vi "UHR-Fleezers Control (host) - Lorentz v2.vi"() -> ()   [LabVIEW 2014]
uses:
  <vilib>/rvi/interface/nirviMethod/nirviMethod.xnode
  <vilib>/rvi/interface/nirviCloseFPGA/nirviCloseFPGA.xnode
  <vilib>/express/express analysis/Spectral/XNode/ExpressSpectralMeasurementsBlockNode.xnode
  <vilib>/rvi/interface/nirviReadWriteControl/nirviReadWriteControl.xnode
  <vilib>/Analysis/NI_AALBase.lvlib
  <vilib>/express/express analysis/Spectral/Block/exnSpectralBlock spectral measurements PSD poly.vi
  <vilib>/rvi/interface/nirviOpenFPGA/nirviOpenFPGA.xnode
  <vilib>/Platform/TimedLoop/XDataNode/XDataNode.xnode
  <vilib>/Platform/TimedLoop/XDataNode/nitl_modes.ctl
  <vilib>/Platform/TimedLoop/XDataNode/XDNodeRunTimeDep.lvlib
  <vilib>/Platform/TimedLoop/XDataNode/wakeup.ctl
  <vilib>/Platform/TimedLoop/XDataNode/timing_clust.ctl
  <vilib>/Utility/miscctls.llb/LVPoint32TypeDef.ctl
  <vilib>/userdefined/High Color/nirio_resource_hc.ctl
  openfpgaref.8.6.ctl
  <vilib>/Utility/miscctls.llb/LVMinMaxIncTypeDef.ctl
  <vilib>/Instr/_visa.llb/VISA Configure Serial Port (Instr).vi
  <vilib>/Analysis/baseanly.llb/Mean (DBL).vi
  Duncan Nall/Fluorescence simulation/Global for fluorescence simulation mean (30 samples), (power series).vi
  <vilib>/vision/Avi.llb/IMAQ AVI2 Refnum.ctl
  <vilib>/gmath/NI_Gmath.lvlib
  <vilib>/addons/database/NI_Database_API.lvlib
  uFLUX control_v2/uFLUX control_v2/Pressure Control/Pressure Control.lvclass
  uFLUX control_v2/uFLUX control_v2/TTL/TTL.lvclass
  uFLUX control_v2/uFLUX control_v2/Pressure Control/Pressure Control Config.ctl
  <vilib>/rvi/errors/niLvFpgaMergeErrorWithErrorCode.vi
  UHR-Fleezers Control (fpga) - Lorentz 1.vi
  <vilib>/addons/database/Connection.llb/DB Tools Open Connec (Path).vi
  <vilib>/Waveform/WDTOps.llb/WDT Index Channel DBL.vi
  <vilib>/Waveform/WDTOps.llb/WDT Append Waveforms DBL.vi
  <vilib>/sound2/lvsound2.llb/Sound Output Write (DBL Single).vi
  <vilib>/express/express analysis/Spectral/Block/exnSpectralBlock spectral measurements PSD WFM.vi
  FPGA Bitfiles/UHR-FleezersInst_FPGATarget_UHR-FleezersCont_eGrpOyvbXfI.lvbitx
  <vilib>/addons/database/Connection.llb/Conn ObjectReference.ctl
  <vilib>/sound2/lvsound2.llb/Sampling Mode.ctl
  <vilib>/sound2/lvsound2.llb/Sound Data Format.ctl
panel:
  in  "Save Event Log?":bool=TRUE
  in  "Stop saving data + video":bool
  in  "Start saving data + video":bool
  in  "Bead diameter":dbl=800.0
  in  "Channel 1 Buffer":string
  in  "DNA Construct":string="oligo binding"
  in  "Title":string="testing database"
  in  "Name":string="test name"
  out "Total Time (s) 2":dbl=60.0
  in  "Start Saving":bool
  in  "Comment (data description)":string="testing confocal setup"
  out "Calibrating Trap...":bool
  in  "N sets to save":u32=200 caption="N Sets"
  in  "Save N Sets":bool
  out "Save file name":path=path "P:/Data/160111/160111_031.dat"
  in  "Save ave N":dbl=100.0 caption="Averaging Factor"
  out "Saving...":bool
  in  "Stop Saving":bool
  out "Progress":u16(slide) scale=0.0..100.0
  out "Save Data Rate (Hz)":dbl=666.6666666666667 caption="Rate (Hz)" format="%#_6p"
  out "Save Data Period (s)":dbl=0.0014999999999999998 caption="Period (s)" format="%#_6p"
  in  "Channel 2 Buffer":string="NA"
  in  "Channel 3 Buffer":string="NA"
  out "Read offset current":string(combo)
  out "PSD Y Sum":dbl[](array[numeric])
  out "log file ref":refnum<file>
  out "AL Running":bool
  in  "AL Delay (s)":u32
  in  "Stop assembly line":bool
  in  "Cy5 Fl.  Thresh. (kHz)":dbl=24.5
  in  "Cy3 Fl.  Thresh. (kHz)":dbl=19.0
  in  "Get Fluorophore":bool
  in  "X or Y?":bool=TRUE
  out "Red Fluorophore":bool
  out "Green Fluorophore":bool
  in  "Numeric":dbl
  in  "stop":bool
  in  "Start assembly line":bool
  out "Sigma/Mean 3":dbl=nan caption="Sigma/Mean" format="%#_2g"
  out "Rate sigma (Hz) 3":dbl=-0.0 caption="Sigma (Hz)" format="%0.2f"
  out "APD 3 Rate (Hz)":dbl=nan format="%#_3p"
  out "HP3 Flush Time (s)":dbl=90.0
  out "HP1 Flush Time (s)":dbl=60.0
  out "TTrig":cluster{dbl, dbl}(graph)
  in  "Sample Channel\nFlow":bool
  in  "Inject Pump 1":bool
  in  "Inject Pump 3":bool
  in  "Pump 1 contents":string="Bottom: DNA beads" caption="Contents"
  in  "Pump 3 contents":string="Top: ADig beads" caption="Contents"
  out "Time (s)":dbl=5.700284999999999
  in  "Index":dbl=1.0 caption="Save File Index" min=1.0 step=1.0
  in  "Scripts":T1(tab)
  in  "Calibrate after bead 2?":bool
  in  "Number of Pulses for bead 2":i32
  in  "Number of pulses for Bead 1":i32
  in  "Get New Beads":bool
  in  "Fixed Traps Data\nScript":bool
  in  "Dump spot flow on?":bool=TRUE caption="Flow ON?"
  in  "Daq spot flow on":bool=TRUE caption="Flow ON?"
  in  "Cap 1 Samp Flow ON":bool=TRUE
  in  "Cap 2 Samp Flow ON":bool=TRUE
  in  "Got Bead 2":bool
  in  "Got Bead 1":bool
  in  "Cap 2 Flow ON":bool=TRUE
  in  "Cap 1 Flow ON":bool=TRUE
  in  "Cap 2 T ON":bool=TRUE
  in  "Move Cap. 2 (ADig Top)":bool
  in  "Move Cap. 1 (DNA Bottom)":bool
  in  "Cal/Data Acq. Spot":bool
  in  "Dump Beads":bool
  in  "Cap 1 T ON":bool=TRUE
  in  "Force FB Data\nScript":bool
  in  "Cap. 2 BD T1?\n(ADig T1, DNA T2)":bool
  in  "Flow Cal":bool
  in  "Pulse Duration (0-100 ms)":dbl=10.0
  in  "Number of pulses For laminar flow":i32=1
  in  "Vent pressure":bool=TRUE
  in  "Pressure Up":bool=TRUE
  in  "Pressure Down":bool=TRUE
  in  "Active cal after cal?":bool
  in  "Fish after cal?":bool
  in  "Flow ON during cal?":bool
  in  "Offset 2 Set":dbl=2.0
  in  "Offset 1 Set":dbl
  in  "Cal @ (MHz)":dbl=14.0
  in  "W/ Offset 1":bool=TRUE
  in  "Offset 1 Start (MHz)":dbl=10.0
  in  "W/ Offset 2":bool
  in  "Offset 2 Start (MHz)":dbl=16.0
  in  "Cal Stage Position":i32=3
  in  "Flow based calibration?":bool
  in  "Lumicks Flow During Calibration":bool
  in  "Only check fixed trap T2":bool
  in  "Flow ON after\ntether testing?":bool
  in  "Flow ON during \nfishing?":bool
  in  "Fish again after \nraster break?":bool
  in  "Furthest Delta (MHz)":dbl=15.0 step=0.25
  in  "Green ON During Raster":bool
  in  "Move to Delta 2 (MHz)":dbl=12.3
  in  "Attempt Limit":dbl=20.0 caption="Limit"
  out "Attempts":dbl=10.0
  in  "Wait Before Save (s)":u32=1
  in  "Closest Delta (MHz)":dbl=8.0 step=0.25
  in  "Stop F (pN)":dbl=3.0
  in  "Then...":string(combo)="5"
  in  "Move to Delta 1 (MHz)":dbl=10.0
  in  "Tether Alarm?":bool=TRUE
  out "Tether":bool
  in  "TA Cancel Save?":bool
  in  "TA Green Off?":bool
  in  "Raster Set Upon Tether":u32=5
  in  "Save at end (5, 6)":bool
  in  "Stop Fishing When Tether":bool=TRUE
  in  "Delay before dipping (s)":dbl=5.0
  in  "Start dipping after?":bool
  in  "Green ON after FB ON?":bool
  in  "Remove Action Offset":bool
  in  "Stage Position To Establish FB":i32=3
  in  "Trap Trig Fl.":bool
  in  "Starting \nTrap Delta (MHz)":dbl=15.25
  in  "Trap Delta Before Moving":dbl=13.0
  in  "Wait (s)":u32=1
  in  "Green ON":bool
  in  "Start dipping after?":bool=TRUE
  in  "Fixed Traps Trap Delta (MHz)":dbl=15.25 caption="Trap Delta (MHz)"
  out "TTrig Fin Thresh (nm)":dbl
  out "TTrig Sig (nm)":dbl
  out "Threshold stored (nm)":dbl
  in  "Neg. TTrig FPGA":bool=TRUE
  in  "Test ttrig":bool
  in  "Trap Trig. (FPGA)":bool=TRUE
  out "Initializing":bool
  in  "Reinitialize":bool
  out "Triggered":bool
  out "Waiting":bool
  in  "Trap Trig. Fl.":bool
  in  "Wait to get offset (n)":u32=10
  in  "Threshold (nm)":dbl=15.0
  in  "Fl. ON time (n)":i32=90
  out "T1 x pos data":dbl[](array[numeric])
  out "max value":dbl=-0.9003514563721442
  out "min value":dbl=-1.184251119672945
  in  "Mean T1 Position\nto compare (nm)":dbl caption="Mean T1 for Comparison (nm)" format="%0.2f"
  out "mean":dbl=-1.0423012880225446 format="%0.2f"
  out "standard\ndeviation":dbl=0.2007473770965739 format="%0.2f"
  out "TTrig Sig (Int)":i64
  out "TTrig Fin Thresh (Int)":i64
  in  "FB Trig Integrate":u32=1
  in  "Green ON\nafter start\nreturn?":bool
  in  "Green delay after \nstart return (s)":dbl
  out "Dwell Time (s)":dbl
  in  "FB OFF when \nflow ON":bool
  in  "Flow ON \nduring return\nfrom dip?":bool=TRUE
  in  "Flow ON\nduring daq?":bool=TRUE
  in  "Flow ON\nduring dip?":bool=TRUE
  in  "Cancel dwell":bool
  in  "Pause dwell":bool
  in  "Dwell Duration (s)":i32=45
  in  "Green ON\nbefore dip?":bool
  in  "Cont. Repeat Dipping?":bool=TRUE
  in  "Dipping Delta (MHz)":dbl=15.0
  in  "Move trap \nbefore dip move?":bool
  in  "Save data after return?":bool
  in  "Green ON \nafter return?":bool=TRUE
  in  "Dip Trap Delta 2 (MHz)":dbl=15.0
  in  "Move trap after return?":bool
  in  "Dip Duration (s)":i32=15
  in  "Dip for Protein":bool
  in  "Dip Stage \nPosition":i32=5
  in  "Return Stage \nPosition":i32=3
  out "Dip Time (s)":i32=16
  out "Dip #":i32=5
  in  "Y change (mm)":dbl=-3.0
  in  "Profile":bool
  out "Current Position":cluster{dbl, dbl, dbl}={1.6, 0.50781, -0.0311}
  in  "Shift confocal":bool
  in  "Auto F Reset":bool
  in  "Yank when?":bool
  in  "Yank to which?":bool
  in  "Yank to SP":dbl[](array[numeric])=[-0.128, -0.158, -0.183, -0.21, -0.01, -0.0319, -0.094, -0.143]
  in  "APD to Watch":bool
  out "Duration (s)":dbl=8.399999999999977
  in  "Action":string(combo)="Yank"
  in  "Fl. Triggered...":bool
  in  "Fl. Delta Thresh. (kHz)":dbl=0.14
  out "Waiting":bool
  out "Fl. High":bool
  in  "N pts to average":u16=6
  in  "Yank Delay (s)":dbl=3.0
  in  "Yank to Trap Delta (MHz)":dbl[](array[numeric])=[16.3, 15.85, 14.85]
  in  "N Array El":u8=4 min=1 step=1
  in  "Random Choice":bool=TRUE
  in  "Force Yank":bool
  in  "Reset Force":bool
  in  "N Steps":dbl=20.0
  in  "Step Size (nm)":dbl=0.34
  in  "Save ave factor":dbl=1.0
  in  "Take Stepping Data":bool
  out "Sigma/Mean 2":dbl=nan caption="Sigma/Mean" format="%#_2g"
  out "Rate sigma (Hz) 2":dbl=-0.0 caption="Sigma (Hz)" format="%0.2f"
  out "APD 2 Rate (Hz)":dbl=nan format="%#_3p"
  out "Primary Video Display":T2(plugin-control)
  out "Waveform Graph":dbl[](graph)=[25.0, 1151.0, 841.0, 408.0, 301.0, 290.0, 352.0, 294.0, 340.0, 282.0, 211.0, 161.0, 111.0, 35.0, 21.0, 13.0, 7.0, 8.0, 6.0, 2.0, 6.0, 11.0, 2.0, 3.0, 7.0, 8.0, 12.0, 13.0, 20.0, 53.0, 62.0, 57.0, 60.0, 49.0, 37.0, 25.0, 16.0, 5.0, 4.0, 4.0, 1.0, 1.0, 1.0, 4.0, 7.0, 9.0, 12.0, 16.0, 28.0, 31.0, 50.0, 54.0, 55.0, 47.0, 50.0, 30.0, 9.0, 10.0, 4.0, 3.0, 3.0, 0.0, 1.0, 2.0, 1.0, 3.0, 9.0, 10.0, 32.0, 32.0, 86.0, 115.0, 183.0, 243.0, 350.0, 369.0, 337.0, 307.0, 224.0, 155.0] caption="APD Line Scan"
  out "Messages":string="14:51\tUHR-Fleezers ready.\r"
  in  "APD Ave N":dbl=20.0
  out "Int. Time (s)":dbl
  in  "Stop All":bool=TRUE
  out "Sigma/Mean":dbl=nan format="%#_2g"
  out "Rate sigma (Hz)":dbl=-0.0 caption="Sigma (Hz)" format="%0.2f"
  in  "Tab Control 6":T3(tab)
  in  "APD 3 Offset":dbl
  in  "APD 2 Offset":dbl
  in  "APD 1 Offset":dbl
  out "RMS (Ang)":dbl=nan format="%_2g"
  in  "Bead Sep. Int. Time (s)":dbl=3.0 caption="Int. Time (s)"
  in  "Below (kHz)":dbl=1.0
  in  "Above (kHz)":dbl=2.0
  in  "Adjust Scale\nto Mean":bool
  in  "Remove Offset":bool
  in  "Offset (nm)":dbl format="%#_3g"
  out "Mean":dbl=nan caption="Mean (pN)" format="%#_3g"
  out "Force":waveform(dbl)[](graph)=[{"t0"=timestamp(0 s since 1904-01-01), "dt"=0.15, "Y"=[], "attributes"=variant("NI_ChannelName"=variant(string "T1 X"))}, {"t0"=timestamp(0 s since 1904-01-01), "dt"=0.15, "Y"=[], "attributes"=variant("NI_ChannelName"=variant(string "T2 X"))}, {"t0"=timestamp(0 s since 1904-01-01), "dt"=0.15, "Y"=[], "attributes"=variant("NI_ChannelName"=variant(string "T1 X"))}]
  out "APD Chart":waveform(dbl)[](graph)=[{"t0"=timestamp(0 s since 1904-01-01), "dt"=0.15, "Y"=[], "attributes"=variant("NI_ChannelName"=variant(string "APD 1"))}, {"t0"=timestamp(0 s since 1904-01-01), "dt"=0.15, "Y"=[], "attributes"=variant("NI_ChannelName"=variant(string "APD 2"))}, {"t0"=timestamp(0 s since 1904-01-01), "dt"=0.15, "Y"=[], "attributes"=variant("NI_ChannelName"=variant(string "APD 3"))}]
  in  "Calibration":u16(ring)=2 items=["None", "Position", "Force"]
  out "T1 X":dbl=nan caption="T1 X (pN)" format="%0.2f"
  out "T2 X":dbl=nan caption="T2 X (pN)" format="%0.2f"
  out "Bead Separation":waveform(dbl)(graph)={"t0"=timestamp(0 s since 1904-01-01), "dt"=0.15, "Y"=[], "attributes"=variant("NI_ChannelName"=variant(string "T1 X"))}
  out "Bead Mean (nm)":dbl=nan caption="Mean (nm)" format="%0.2f"
  out "Difference":dbl=nan caption="Difference (pN)" format="%.2g"
  out "Confocal Y 2 (V)":dbl=6.809280068361465
  out "Confocal X 2 (V)":dbl=0.7223435163426621
  out "Confocal Y 1 (V)":dbl=5.709081392864773
  out "Confocal X 1 (V)":dbl=4.827825251014741
  in  "Set High F Confocal Spot (X-Y)":bool
  in  "Take Detection Laser\nImage":bool
  out "APD 2":T2(plugin-control) caption="APD 2 (Cy5)"
  in  "Flip Green Filter":bool
  in  "Set X Only":bool
  in  "Set Y Only":bool
  out "APD 1":T2(plugin-control) caption="APD 1 (Cy3)"
  out "Detection Laser Y":T2(plugin-control)
  out "Pointer Y (V)":dbl=4.837472762230294 format="%_3g"
  out "Pointer X (V)":dbl=8.31425977355266 format="%_3g"
  in  "Set Confocal Spot (X-Y)":bool
  out "Detection Laser X":T2(plugin-control)
  out "APD 3":T2(plugin-control) caption="APD 3 (Cy2)"
  in  "Display Saved Data":string(combo)
  out "Saved trap pos":dbl[](graph)
  out "Saved APD":dbl[][](graph)=[[126.66666666666667, 113.33333333333334, 126.66666666666667, 113.33333333333334, 80.0, 133.33333333333334, 53.333333333333336, 106.66666666666667, 86.66666666666667, 53.333333333333336, 80.0, 160.0, 113.33333333333334, 100.0, 120.0, 153.33333333333334, 140.0, 93.33333333333334, 106.66666666666667, 133.33333333333334, 113.33333333333334, 100.0, 126.66666666666667, 140.0, 153.33333333333334, 100.0, 60.0, 120.0, 86.66666666666667, 80.0, 100.0, 73.33333333333334, 86.66666666666667, 113.33333333333334, 60.0, 126.66666666666667, 113.33333333333334, 100.0, 113.33333333333334, 113.33333333333334, 93.33333333333334, 86.66666666666667, 146.66666666666669, 86.66666666666667, 126.66666666666667, 80.0, 113.33333333333334, 153.33333333333334, 86.66666666666667, 60.0, 86.66666666666667, 106.66666666666667, 113.33333333333334, 106.66666666666667, 133.33333333333334, 133.33333333333334, 53.333333333333336, 146.66666666666669, 153.33333333333334, 80.0, 73.33333333333334, 113.33333333333334, 100.0, 113.33333333333334, 120.0, 86.66666666666667, 86.66666666666667, 93.33333333333334, 60.0, 80.0, 120.0, 126.66666666666667, 46.66666666666667, 173.33333333333334, 113.33333333333334, 66.66666666666667, 140.0, 113.33333333333334, 53.333333333333336, 86.66666666666667, 46.66666666666667, 80.0, 113.33333333333334, 126.66666666666667, 100.0, 60.0, 93.33333333333334, 80.0, 106.66666666666667, 140.0, 113.33333333333334, 140.0, 93.33333333333334, 106.66666666666667, 93.33333333333334, 86.66666666666667, 140.0, 133.33333333333334, 1760.0, 3533.3333333333335, 380.0, 4466.666666666667, 5073.333333333334, 826.6666666666667, 6466.666666666667, 2680.0, 4713.333333333334, 8260.0, 1026.6666666666667, 8900.0, 8820.0, 1940.0, 10873.333333333334, 4460.0, 5406.666666666667, 9986.666666666668, 1446.6666666666667, 9040.0, 6800.0, 1920.0, 7273.333333333334, 3226.666666666667, 3053.3333333333335, 5526.666666666667, 753.3333333333334, 3440.0, 2600.0, 726.6666666666667, 1993.3333333333335, 973.3333333333334, 0.0, 0.0, 6.666666666666667, 20.0, 6.666666666666667, 0.0, 0.0, 13.333333333333334, 0.0, 13.333333333333334, 6.666666666666667, 0.0, 0.0, 6.666666666666667, 6.666666666666667, 6.666666666666667, 6.666666666666667, 20.0, 0.0, 6.666666666666667, 0.0, 6.666666666666667, 6.666666666666667, 0.0, 0.0, 0.0, 0.0, 0.0, 6.666666666666667, 6.666666666666667, 0.0, 6.666666666666667, 58873.333333333336, 88753.33333333334, 58686.66666666667, 82013.33333333334, 73680.0, 86226.66666666667, 161553.33333333334, 90873.33333333334, 99960.0, 160820.0, 143406.6666666667, 123873.33333333334, 111920.0, 138946.6666666667, 203493.33333333334, 115073.33333333334, 113620.0, 165526.6666666667, 162766.6666666667, 108720.0, 105680.0, 128066.66666666667, 161266.6666666667, 91606.66666666667, 81740.0, 105920.0, 114013.33333333334, 57840.0, 56013.333333333336, 49453.333333333336, 55046.66666666667, 24753.333333333336, 37073.333333333336, 59220.0, 40473.333333333336, 53360.0, 48266.66666666667, 57626.66666666667, 113800.0, 64993.333333333336, 76386.66666666667, 121100.0, 109613.33333333334, 93006.66666666667, 87486.66666666667, 109153.33333333334, 161280.0, 91160.0, 90606.66666666667, 134300.0, 129660.0, 88133.33333333334, 85346.66666666667, 100960.0, 129826.66666666667, 74526.66666666667, 63600.0, 86580.0, 90173.33333333334, 43646.66666666667, 42160.0, 37413.333333333336, 39540.0, 16886.666666666668, 83180.0, 145886.6666666667, 135013.33333333334, 143420.0, 131746.6666666667, 171326.6666666667, 260526.6666666667, 152053.33333333334, 159300.0, 237413.33333333334, 234720.0, 179213.33333333334, 168473.33333333334, 213053.33333333334, 275106.6666666667, 166913.33333333334, 163233.33333333334, 234900.0, 240626.6666666667, 161813.33333333334, 156160.0, 194220.0, 241986.6666666667, 141060.0, 130106.66666666667, 178380.0, 181720.0, 101760.0, 97240.0, 91920.0, 106166.66666666667, 53620.0, 49766.66666666667, 69306.66666666667, 76120.0, 85406.66666666667, 80873.33333333334, 111693.33333333334, 191113.33333333334, 113333.33333333334, 122166.66666666667, 187080.0, 194293.33333333334, 142746.6666666667, 138233.33333333334, 178420.0, 243293.33333333334, 143806.6666666667, 139293.33333333334, 202140.0, 213406.6666666667, 138013.33333333334, 136020.0, 165513.33333333334, 212093.33333333334, 120806.66666666667, 109833.33333333334, 149353.33333333334, 148793.33333333334, 77393.33333333334, 77113.33333333334, 69493.33333333334, 77660.0, 33440.0, 50560.0, 68646.66666666667, 74726.66666666667, 84220.0, 78213.33333333334, 109353.33333333334, 188906.6666666667, 110473.33333333334, 123720.0, 187960.0, 194106.6666666667, 144266.6666666667, 138713.33333333334, 174200.0, 242460.0, 143686.6666666667, 141326.6666666667, 201426.6666666667, 211853.33333333334, 138133.33333333334, 136433.33333333334, 162713.33333333334, 215760.0, 122100.0, 109560.0, 151720.0, 151620.0, 78946.66666666667, 79433.33333333334, 68566.66666666667, 82966.66666666667, 37260.0, 14106.666666666668, 13780.0, 19180.0, 19686.666666666668, 20360.0, 33320.0, 69573.33333333334, 39166.66666666667, 48846.66666666667, 84226.66666666667, 91106.66666666667, 62666.66666666667, 58206.66666666667, 74120.0, 110460.0, 58186.66666666667, 61666.66666666667, 88013.33333333334, 91280.0, 58646.66666666667, 58420.0, 65173.333333333336, 87826.66666666667, 47933.333333333336, 41393.333333333336, 49720.0, 50586.66666666667, 20986.666666666668, 21160.0, 13453.333333333334, 16726.666666666668, 6206.666666666667, 67173.33333333334, 100193.33333333334, 104320.0, 110186.66666666667, 103286.66666666667, 139606.6666666667, 222940.0, 130420.0, 139753.33333333334, 209046.6666666667, 211860.0, 159173.33333333334, 152006.6666666667, 192673.33333333334, 259866.6666666667, 154100.0, 153553.33333333334, 217093.33333333334, 223493.33333333334, 147993.33333333334, 144046.6666666667, 177720.0, 223973.33333333334, 129053.33333333334, 117240.0, 159020.0, 157046.6666666667, 83680.0, 79880.0, 72200.0, 86860.0, 38986.66666666667, 11033.333333333334, 11433.333333333334, 18180.0, 21460.0, 19020.0, 35926.66666666667, 65173.333333333336, 37820.0, 45606.66666666667, 70533.33333333334, 83633.33333333334, 50833.333333333336, 52286.66666666667, 69380.0, 100033.33333333334, 57246.66666666667, 50233.333333333336, 73880.0, 81306.66666666667, 52020.0, 50640.0, 64780.0, 78986.66666666667, 45466.66666666667, 35400.0, 47693.333333333336, 45946.66666666667, 18393.333333333336, 16966.666666666668, 12926.666666666668, 15080.0, 5193.333333333334, 7446.666666666667, 7086.666666666667, 13886.666666666668, 14406.666666666668, 15820.0, 27906.666666666668, 45180.0, 27386.666666666668, 31680.0, 45973.333333333336, 65326.66666666667, 42586.66666666667, 42646.66666666667, 59326.66666666667, 73720.0, 44526.66666666667, 39353.333333333336, 56040.0, 66106.66666666667, 40246.66666666667, 39933.333333333336, 54113.333333333336, 59526.66666666667, 33786.66666666667, 27826.666666666668, 33466.66666666667, 38540.0, 14500.0, 13646.666666666668, 11393.333333333334, 10433.333333333334, 3666.666666666667, 7286.666666666667, 7800.0, 11813.333333333334, 14140.0, 14900.0, 25013.333333333336, 44160.0, 27293.333333333336, 34553.333333333336, 47473.333333333336, 64253.333333333336, 38960.0, 41173.333333333336, 51546.66666666667, 64260.0, 38813.333333333336, 37706.66666666667, 52513.333333333336, 61353.333333333336, 36746.66666666667, 34513.333333333336, 44786.66666666667, 49726.66666666667, 28846.666666666668, 21580.0, 30246.666666666668, 30433.333333333336, 12300.0, 11606.666666666668, 8053.333333333334, 6646.666666666667, 3166.666666666667, 7313.333333333334, 6826.666666666667, 9246.666666666668, 12060.0, 10813.333333333334, 21320.0, 39206.66666666667, 24040.0, 28600.0, 42253.333333333336, 59766.66666666667, 31160.0, 34020.0, 43793.333333333336, 54166.66666666667, 33813.333333333336, 33253.333333333336, 39600.0, 51773.333333333336, 31746.666666666668, 29406.666666666668, 39226.66666666667, 43393.333333333336, 25960.0, 21453.333333333336, 25940.0, 32280.0, 12853.333333333334, 10880.0, 7473.333333333334, 7173.333333333334, 2920.0, 56953.333333333336, 85960.0, 58406.66666666667, 90333.33333333334, 84813.33333333334, 120433.33333333334, 207333.33333333334, 121233.33333333334, 137100.0, 211380.0, 212946.6666666667, 175960.0, 158733.33333333334, 214973.33333333334, 269733.3333333334, 169720.0, 163193.33333333334, 235040.0, 255906.6666666667, 166186.6666666667, 159446.6666666667, 215633.33333333334, 244666.6666666667, 153406.6666666667, 147000.0, 191020.0, 219800.0, 124920.0, 124533.33333333334, 147293.33333333334, 157046.6666666667, 88060.0, 54086.66666666667, 70540.0, 76433.33333333334, 81826.66666666667, 85986.66666666667, 113520.0, 176380.0, 112013.33333333334, 123620.0, 173073.33333333334, 198520.0, 139326.6666666667, 135673.33333333334, 187406.6666666667, 227553.33333333334, 144433.33333333334, 140100.0, 190633.33333333334, 223760.0, 137513.33333333334, 134286.6666666667, 176153.33333333334, 199046.6666666667, 119846.66666666667, 108193.33333333334, 137506.6666666667, 160513.33333333334, 75686.66666666667, 77973.33333333334, 74446.66666666667, 71320.0, 34140.0, 35486.66666666667, 47333.333333333336, 55853.333333333336, 61040.0, 57560.0, 86853.33333333334, 140953.33333333334, 90080.0, 99880.0, 142580.0, 178360.0, 121720.0, 121386.66666666667, 156453.33333333334, 196960.0, 125066.66666666667, 121120.0, 169926.6666666667, 196686.6666666667, 121786.66666666667, 118093.33333333334, 158286.6666666667, 173840.0, 106106.66666666667, 95486.66666666667, 115780.0, 135840.0, 60906.66666666667, 60800.0, 53900.0, 55026.66666666667, 26106.666666666668, 48733.333333333336, 70033.33333333334, 9786.666666666668, 97153.33333333334, 106946.66666666667, 50066.66666666667, 162993.33333333334, 135240.0, 169180.0, 240760.0, 115480.0, 279280.0, 243513.33333333334, 170540.0, 246993.33333333334, 239593.33333333334, 217593.33333333334, 267820.0, 139560.0, 262060.0, 222146.6666666667, 136953.33333333334, 206126.6666666667, 159126.6666666667, 109660.0, 153573.33333333334, 16346.666666666668, 100873.33333333334, 53153.333333333336, 9793.333333333334, 29960.0, 11113.333333333334, 36153.333333333336, 44553.333333333336, 9400.0, 65753.33333333334, 72673.33333333334, 46580.0, 121946.66666666667, 122980.0, 150580.0, 206953.33333333334, 111460.0, 250006.6666666667, 218440.0, 173186.6666666667, 227593.33333333334, 227180.0, 205006.6666666667, 243653.33333333334, 130620.0, 242040.0, 198446.6666666667, 133746.6666666667, 186313.33333333334, 140640.0, 91306.66666666667, 124153.33333333334, 15173.333333333334, 76546.66666666667, 35246.66666666667, 8000.0, 18240.0, 6306.666666666667, 100.0, 53.333333333333336, 46.66666666666667, 73.33333333333334, 93.33333333333334, 60.0, 40.0, 53.333333333333336, 106.66666666666667, 106.66666666666667, 60.0, 93.33333333333334, 66.66666666666667, 66.66666666666667, 73.33333333333334, 66.66666666666667, 73.33333333333334, 40.0, 53.333333333333336, 93.33333333333334, 46.66666666666667, 33.333333333333336, 66.66666666666667, 80.0, 33.333333333333336, 73.33333333333334, 80.0, 53.333333333333336, 33.333333333333336, 60.0, 73.33333333333334, 66.66666666666667, 73.33333333333334, 60.0, 106.66666666666667, 80.0, 80.0, 46.66666666666667, 66.66666666666667, 126.66666666666667, 46.66666666666667, 26.666666666666668, 46.66666666666667, 33.333333333333336, 66.66666666666667, 93.33333333333334, 73.33333333333334, 66.66666666666667, 73.33333333333334, 60.0, 53.333333333333336, 80.0, 33.333333333333336, 60.0, 100.0, 80.0, 80.0, 73.33333333333334, 73.33333333333334, 126.66666666666667, 46.66666666666667, 106.66666666666667, 106.66666666666667, 120.0, 113.33333333333334, 93.33333333333334, 93.33333333333334, 66.66666666666667, 100.0, 120.0, 53.333333333333336, 113.33333333333334, 133.33333333333334, 140.0, 53.333333333333336, 160.0, 160.0, 106.66666666666667, 113.33333333333334, 66.66666666666667, 106.66666666666667, 106.66666666666667, 100.0, 146.66666666666669, 173.33333333333334, 120.0, 93.33333333333334, 153.33333333333334, 113.33333333333334, 126.66666666666667, 100.0, 133.33333333333334, 146.66666666666669, 180.0, 126.66666666666667, 126.66666666666667, 126.66666666666667, 93.33333333333334, 126.66666666666667, 93.33333333333334, 120.0, 80.0, 93.33333333333334, 100.0, 73.33333333333334, 146.66666666666669, 100.0, 46.66666666666667, 53.333333333333336, 40.0, 73.33333333333334, 60.0, 80.0, 80.0, 66.66666666666667, 60.0, 53.333333333333336, 80.0, 86.66666666666667, 33.333333333333336, 66.66666666666667, 73.33333333333334, 86.66666666666667, 73.33333333333334, 53.333333333333336, 66.66666666666667, 66.66666666666667, 73.33333333333334, 40.0, 100.0, 46.66666666666667, 46.66666666666667, 86.66666666666667, 53.333333333333336, 66.66666666666667, 60.0, 93.33333333333334, 73.33333333333334, 60.0, 86.66666666666667, 53.333333333333336, 53.333333333333336, 86.66666666666667, 53.333333333333336, 66.66666666666667, 66.66666666666667, 66.66666666666667, 60.0, 100.0, 40.0, 60.0, 40.0, 46.66666666666667, 73.33333333333334, 53.333333333333336, 60.0, 86.66666666666667, 86.66666666666667, 60.0, 46.66666666666667, 33.333333333333336, 86.66666666666667, 106.66666666666667, 60.0, 40.0, 86.66666666666667, 66.66666666666667, 53.333333333333336, 46.66666666666667, 86.66666666666667, 13.333333333333334, 53.333333333333336, 73.33333333333334, 46.66666666666667, 53.333333333333336, 80.0, 86.66666666666667, 40.0, 100.0, 86.66666666666667, 80.0, 53.333333333333336, 66.66666666666667, 60.0, 60.0, 113.33333333333334, 60.0, 60.0, 53.333333333333336, 100.0, 80.0, 53.333333333333336, 73.33333333333334, 86.66666666666667, 73.33333333333334, 53.333333333333336, 73.33333333333334, 113.33333333333334, 100.0, 80.0, 66.66666666666667, 66.66666666666667, 53.333333333333336, 60.0, 86.66666666666667, 73.33333333333334, 120.0, 106.66666666666667, 73.33333333333334, 40.0, 120.0, 86.66666666666667, 66.66666666666667, 113.33333333333334, 120.0, 106.66666666666667, 126.66666666666667, 133.33333333333334, 93.33333333333334, 113.33333333333334, 120.0, 86.66666666666667, 100.0, 106.66666666666667, 160.0, 86.66666666666667, 100.0, 93.33333333333334, 113.33333333333334, 133.33333333333334, 120.0, 93.33333333333334, 140.0, 193.33333333333334, 113.33333333333334, 146.66666666666669, 160.0, 153.33333333333334, 166.66666666666669, 106.66666666666667, 120.0, 133.33333333333334, 126.66666666666667, 140.0, 146.66666666666669, 106.66666666666667, 153.33333333333334, 120.0, 140.0, 153.33333333333334, 126.66666666666667, 113.33333333333334, 86.66666666666667, 166.66666666666669, 126.66666666666667, 73.33333333333334, 93.33333333333334, 66.66666666666667, 113.33333333333334, 80.0, 113.33333333333334, 100.0, 93.33333333333334, 80.0, 86.66666666666667, 100.0, 120.0, 106.66666666666667, 93.33333333333334, 33.333333333333336, 46.66666666666667, 66.66666666666667, 46.66666666666667, 100.0, 53.333333333333336, 80.0, 66.66666666666667, 46.66666666666667, 113.33333333333334, 40.0, 66.66666666666667, 80.0, 46.66666666666667, 93.33333333333334, 86.66666666666667, 66.66666666666667, 93.33333333333334, 53.333333333333336, 53.333333333333336, 73.33333333333334, 86.66666666666667, 86.66666666666667, 66.66666666666667, 73.33333333333334, 73.33333333333334, 100.0, 60.0, 93.33333333333334, 100.0, 100.0, 73.33333333333334, 66.66666666666667, 60.0, 66.66666666666667, 53.333333333333336, 60.0, 73.33333333333334, 86.66666666666667], [213.33333333333334, 226.66666666666669, 213.33333333333334, 226.66666666666669, 253.33333333333334, 226.66666666666669, 233.33333333333334, 260.0, 273.33333333333337, 260.0, 200.0, 253.33333333333334, 166.66666666666669, 360.0, 320.0, 246.66666666666669, 266.6666666666667, 286.6666666666667, 286.6666666666667, 246.66666666666669, 253.33333333333334, 300.0, 273.33333333333337, 266.6666666666667, 300.0, 226.66666666666669, 253.33333333333334, 313.33333333333337, 260.0, 260.0, 266.6666666666667, 260.0, 193.33333333333334, 233.33333333333334, 166.66666666666669, 286.6666666666667, 153.33333333333334, 253.33333333333334, 233.33333333333334, 233.33333333333334, 280.0, 260.0, 240.0, 233.33333333333334, 273.33333333333337, 206.66666666666669, 213.33333333333334, 220.0, 260.0, 233.33333333333334, 226.66666666666669, 233.33333333333334, 233.33333333333334, 233.33333333333334, 246.66666666666669, 340.0, 226.66666666666669, 300.0, 180.0, 246.66666666666669, 280.0, 240.0, 206.66666666666669, 253.33333333333334, 300.0, 346.6666666666667, 193.33333333333334, 233.33333333333334, 280.0, 220.0, 233.33333333333334, 186.66666666666669, 233.33333333333334, 333.33333333333337, 260.0, 300.0, 280.0, 226.66666666666669, 193.33333333333334, 286.6666666666667, 286.6666666666667, 160.0, 206.66666666666669, 213.33333333333334, 166.66666666666669, 133.33333333333334, 233.33333333333334, 226.66666666666669, 220.0, 173.33333333333334, 320.0, 160.0, 253.33333333333334, 213.33333333333334, 220.0, 213.33333333333334, 306.6666666666667, 226.66666666666669, 19306.666666666668, 29680.0, 12346.666666666668, 35300.0, 38120.0, 17440.0, 57573.333333333336, 28773.333333333336, 39006.66666666667, 64260.0, 26566.666666666668, 64213.333333333336, 61346.66666666667, 28220.0, 82460.0, 40420.0, 46246.66666666667, 72966.66666666667, 30100.0, 62320.0, 52406.66666666667, 27553.333333333336, 59713.333333333336, 27826.666666666668, 28046.666666666668, 40320.0, 17220.0, 25506.666666666668, 22033.333333333336, 9633.333333333334, 20320.0, 9173.333333333334, 20.0, 13.333333333333334, 20.0, 20.0, 13.333333333333334, 20.0, 26.666666666666668, 6.666666666666667, 26.666666666666668, 6.666666666666667, 26.666666666666668, 26.666666666666668, 13.333333333333334, 0.0, 6.666666666666667, 6.666666666666667, 6.666666666666667, 26.666666666666668, 6.666666666666667, 20.0, 20.0, 13.333333333333334, 20.0, 13.333333333333334, 6.666666666666667, 13.333333333333334, 20.0, 33.333333333333336, 0.0, 20.0, 13.333333333333334, 20.0, 96213.33333333334, 130313.33333333334, 133393.33333333334, 128360.0, 119980.0, 160973.33333333334, 243486.6666666667, 149433.33333333334, 157460.0, 234966.6666666667, 231206.6666666667, 182833.33333333334, 169606.6666666667, 216926.6666666667, 285993.3333333334, 176700.0, 173080.0, 245840.0, 246286.6666666667, 177780.0, 168513.33333333334, 208560.0, 263140.0, 155893.33333333334, 147433.33333333334, 204820.0, 200546.6666666667, 127813.33333333334, 121360.0, 122180.0, 159686.6666666667, 81033.33333333334, 66793.33333333334, 94580.0, 99453.33333333334, 95206.66666666667, 90006.66666666667, 125846.66666666667, 198633.33333333334, 123060.0, 135780.0, 202600.0, 204633.33333333334, 157606.6666666667, 150320.0, 196040.0, 259426.6666666667, 155840.0, 157280.0, 227493.33333333334, 223600.0, 159526.6666666667, 152953.33333333334, 185380.0, 240293.33333333334, 142593.33333333334, 128820.0, 186833.33333333334, 174900.0, 107406.66666666667, 103086.66666666667, 102613.33333333334, 129273.33333333334, 63633.333333333336, 158246.6666666667, 245193.33333333334, 226953.33333333334, 211880.0, 192906.6666666667, 241386.6666666667, 321380.0, 206973.33333333334, 204106.6666666667, 294333.3333333334, 275686.6666666667, 227206.6666666667, 208973.33333333334, 259193.33333333334, 313313.3333333334, 206873.33333333334, 197540.0, 282626.6666666667, 270973.3333333334, 210066.6666666667, 192160.0, 240906.6666666667, 291760.0, 182280.0, 170986.6666666667, 240666.6666666667, 228960.0, 156886.6666666667, 145633.33333333334, 153526.6666666667, 190126.6666666667, 109666.66666666667, 104646.66666666667, 147686.6666666667, 146873.33333333334, 137380.0, 131966.6666666667, 167960.0, 254460.0, 157160.0, 160973.33333333334, 242520.0, 236586.6666666667, 186280.0, 174686.6666666667, 219760.0, 290853.3333333334, 179640.0, 172266.6666666667, 251453.33333333334, 249353.33333333334, 179380.0, 169913.33333333334, 206593.33333333334, 262626.6666666667, 156706.6666666667, 145526.6666666667, 207286.6666666667, 194933.33333333334, 124120.0, 119393.33333333334, 120300.0, 151526.6666666667, 77506.66666666667, 104253.33333333334, 146366.6666666667, 147980.0, 137553.33333333334, 128880.0, 167726.6666666667, 253086.6666666667, 154206.6666666667, 162140.0, 245486.6666666667, 233593.33333333334, 188993.33333333334, 174393.33333333334, 219360.0, 290146.6666666667, 179166.6666666667, 174406.6666666667, 250226.6666666667, 246286.6666666667, 181386.6666666667, 170373.33333333334, 206040.0, 266446.6666666667, 158640.0, 145686.6666666667, 209873.33333333334, 196900.0, 125340.0, 120680.0, 119860.0, 155273.33333333334, 81173.33333333334, 30920.0, 36713.333333333336, 43700.0, 40893.333333333336, 40493.333333333336, 59600.0, 110340.0, 61220.0, 71953.33333333334, 120226.66666666667, 121833.33333333334, 89173.33333333334, 83393.33333333334, 108586.66666666667, 154200.0, 84166.66666666667, 88626.66666666667, 130120.0, 130746.66666666667, 88160.0, 85880.0, 96560.0, 131640.0, 72326.66666666667, 64640.0, 84726.66666666667, 80920.0, 41713.333333333336, 40280.0, 30386.666666666668, 43366.66666666667, 19026.666666666668, 128320.0, 187026.6666666667, 181580.0, 166760.0, 158160.0, 200633.33333333334, 285580.0, 177046.6666666667, 179473.33333333334, 266353.3333333334, 249680.0, 203606.6666666667, 188913.33333333334, 239940.0, 305693.3333333334, 193740.0, 189240.0, 266213.3333333334, 258260.0, 194080.0, 179180.0, 224873.33333333334, 278553.3333333334, 167553.33333333334, 157926.6666666667, 220493.33333333334, 205980.0, 135960.0, 125620.0, 131100.0, 168100.0, 89580.0, 25513.333333333336, 31113.333333333336, 40406.66666666667, 40626.66666666667, 36613.333333333336, 60826.66666666667, 100600.0, 60713.333333333336, 67393.33333333334, 104773.33333333334, 117666.66666666667, 80093.33333333334, 77920.0, 101926.66666666667, 148680.0, 85886.66666666667, 78586.66666666667, 116246.66666666667, 121526.66666666667, 79166.66666666667, 78033.33333333334, 98053.33333333334, 122046.66666666667, 72553.33333333334, 57700.0, 82520.0, 76866.66666666667, 37973.333333333336, 35720.0, 31800.0, 39053.333333333336, 17473.333333333336, 18193.333333333336, 20706.666666666668, 33580.0, 31086.666666666668, 33653.333333333336, 51180.0, 78246.66666666667, 48320.0, 54166.66666666667, 79606.66666666667, 101820.0, 69846.66666666667, 68853.33333333334, 99373.33333333334, 127460.0, 75840.0, 69566.66666666667, 98600.0, 112866.66666666667, 72566.66666666667, 70613.33333333334, 90173.33333333334, 107053.33333333334, 61940.0, 51826.66666666667, 68506.66666666667, 74380.0, 34840.0, 33393.333333333336, 29593.333333333336, 34326.66666666667, 13506.666666666668, 17120.0, 22613.333333333336, 31253.333333333336, 29940.0, 31753.333333333336, 47793.333333333336, 78366.66666666667, 48673.333333333336, 56566.66666666667, 80920.0, 98320.0, 62986.66666666667, 65920.0, 83973.33333333334, 111540.0, 67986.66666666667, 64713.333333333336, 94500.0, 104106.66666666667, 65900.0, 59520.0, 77213.33333333334, 93526.66666666667, 52420.0, 43020.0, 63060.0, 60966.66666666667, 30360.0, 28566.666666666668, 23166.666666666668, 23486.666666666668, 11100.0, 17326.666666666668, 20520.0, 23840.0, 27073.333333333336, 26006.666666666668, 39713.333333333336, 68213.33333333334, 43593.333333333336, 49160.0, 71686.66666666667, 89506.66666666667, 54606.66666666667, 56260.0, 75280.0, 96480.0, 59406.66666666667, 63653.333333333336, 76406.66666666667, 95853.33333333334, 58326.66666666667, 54013.333333333336, 71726.66666666667, 82806.66666666667, 47393.333333333336, 41413.333333333336, 54773.333333333336, 64133.333333333336, 29606.666666666668, 26393.333333333336, 21633.333333333336, 24186.666666666668, 10293.333333333334, 118740.0, 183966.6666666667, 139800.0, 165386.6666666667, 152620.0, 185166.6666666667, 296520.0, 174680.0, 185060.0, 283866.6666666667, 247580.0, 229666.6666666667, 201686.6666666667, 251233.33333333334, 315786.6666666667, 205353.33333333334, 198786.6666666667, 285313.3333333334, 274366.6666666667, 213920.0, 194793.33333333334, 258846.6666666667, 291626.6666666667, 194853.33333333334, 188133.33333333334, 252100.0, 267853.3333333334, 175740.0, 172073.33333333334, 205280.0, 227513.33333333334, 141106.6666666667, 109353.33333333334, 143866.6666666667, 150800.0, 134660.0, 133820.0, 172366.6666666667, 244873.33333333334, 159820.0, 167986.6666666667, 235453.33333333334, 244133.33333333334, 182600.0, 173820.0, 231273.33333333334, 277620.0, 182080.0, 176600.0, 244873.33333333334, 261346.6666666667, 176306.6666666667, 168886.6666666667, 218933.33333333334, 257460.0, 159533.33333333334, 147606.6666666667, 199980.0, 214526.6666666667, 125013.33333333334, 122186.66666666667, 135826.6666666667, 151093.33333333334, 83226.66666666667, 76973.33333333334, 108360.0, 118800.0, 108813.33333333334, 102306.66666666667, 142220.0, 208700.0, 132333.33333333334, 140100.0, 201273.33333333334, 224186.6666666667, 162226.6666666667, 159760.0, 201726.6666666667, 251826.6666666667, 162366.6666666667, 156046.6666666667, 223600.0, 239393.33333333334, 160533.33333333334, 152213.33333333334, 203166.6666666667, 234453.33333333334, 144620.0, 133780.0, 176520.0, 189106.6666666667, 105506.66666666667, 104413.33333333334, 108293.33333333334, 125186.66666666667, 68133.33333333334, 103080.0, 159293.33333333334, 39900.0, 198566.6666666667, 195760.0, 117920.0, 255900.0, 215660.0, 236506.6666666667, 312120.0, 179366.6666666667, 333826.6666666667, 293900.0, 231506.6666666667, 284140.0, 286500.0, 271266.6666666667, 307406.6666666667, 201493.33333333334, 306020.0, 277173.3333333334, 194313.33333333334, 259446.6666666667, 225940.0, 177893.33333333334, 237920.0, 55133.333333333336, 184993.33333333334, 134946.6666666667, 35340.0, 108646.66666666667, 50286.66666666667, 77580.0, 108060.0, 34373.333333333336, 151060.0, 149580.0, 107500.0, 211666.6666666667, 203433.33333333334, 218633.33333333334, 278293.3333333334, 172440.0, 312793.3333333334, 277720.0, 233553.33333333334, 273053.3333333334, 289240.0, 263553.3333333334, 293613.3333333334, 190406.6666666667, 295693.3333333334, 260880.0, 191740.0, 239260.0, 210906.6666666667, 155006.6666666667, 204133.33333333334, 48033.333333333336, 154406.6666666667, 102913.33333333334, 32260.0, 77780.0, 35800.0, 933.3333333333334, 906.6666666666667, 1000.0, 953.3333333333334, 966.6666666666667, 893.3333333333334, 1046.6666666666667, 873.3333333333334, 906.6666666666667, 960.0, 1000.0, 873.3333333333334, 820.0, 920.0, 913.3333333333334, 860.0, 1073.3333333333335, 953.3333333333334, 973.3333333333334, 933.3333333333334, 1100.0, 846.6666666666667, 966.6666666666667, 1026.6666666666667, 980.0, 980.0, 846.6666666666667, 1013.3333333333334, 933.3333333333334, 1000.0, 900.0, 993.3333333333334, 1053.3333333333335, 900.0, 806.6666666666667, 880.0, 953.3333333333334, 866.6666666666667, 966.6666666666667, 946.6666666666667, 833.3333333333334, 820.0, 880.0, 1013.3333333333334, 940.0, 833.3333333333334, 753.3333333333334, 846.6666666666667, 886.6666666666667, 946.6666666666667, 900.0, 940.0, 840.0, 1026.6666666666667, 1126.6666666666667, 980.0, 1066.6666666666667, 920.0, 1233.3333333333335, 1160.0, 1160.0, 1106.6666666666667, 1320.0, 1226.6666666666667, 1326.6666666666667, 1020.0, 1246.6666666666667, 1320.0, 1353.3333333333335, 1446.6666666666667, 1373.3333333333335, 1533.3333333333335, 1513.3333333333335, 1560.0, 1600.0, 1626.6666666666667, 1620.0, 1606.6666666666667, 1673.3333333333335, 1766.6666666666667, 1720.0, 1793.3333333333335, 1873.3333333333335, 1786.6666666666667, 1880.0, 1953.3333333333335, 1600.0, 1753.3333333333335, 1720.0, 1700.0, 1726.6666666666667, 1633.3333333333335, 1453.3333333333335, 1446.6666666666667, 1340.0, 1213.3333333333335, 1353.3333333333335, 1493.3333333333335, 1333.3333333333335, 1280.0, 1306.6666666666667, 1313.3333333333335, 1240.0, 1133.3333333333335, 1086.6666666666667, 1106.6666666666667, 1153.3333333333335, 1073.3333333333335, 1066.6666666666667, 873.3333333333334, 933.3333333333334, 993.3333333333334, 1040.0, 1020.0, 1006.6666666666667, 1126.6666666666667, 840.0, 840.0, 826.6666666666667, 853.3333333333334, 980.0, 960.0, 966.6666666666667, 933.3333333333334, 853.3333333333334, 940.0, 900.0, 886.6666666666667, 893.3333333333334, 920.0, 1053.3333333333335, 860.0, 993.3333333333334, 966.6666666666667, 960.0, 840.0, 953.3333333333334, 953.3333333333334, 933.3333333333334, 866.6666666666667, 986.6666666666667, 820.0, 866.6666666666667, 1120.0, 806.6666666666667, 933.3333333333334, 993.3333333333334, 1100.0, 946.6666666666667, 966.6666666666667, 1013.3333333333334, 1086.6666666666667, 1173.3333333333335, 833.3333333333334, 966.6666666666667, 920.0, 1133.3333333333335, 920.0, 920.0, 833.3333333333334, 940.0, 893.3333333333334, 853.3333333333334, 933.3333333333334, 933.3333333333334, 873.3333333333334, 980.0, 833.3333333333334, 960.0, 953.3333333333334, 800.0, 813.3333333333334, 906.6666666666667, 913.3333333333334, 920.0, 1013.3333333333334, 966.6666666666667, 846.6666666666667, 846.6666666666667, 920.0, 933.3333333333334, 853.3333333333334, 886.6666666666667, 826.6666666666667, 813.3333333333334, 873.3333333333334, 726.6666666666667, 973.3333333333334, 960.0, 940.0, 926.6666666666667, 820.0, 813.3333333333334, 933.3333333333334, 733.3333333333334, 940.0, 880.0, 1073.3333333333335, 1060.0, 960.0, 940.0, 886.6666666666667, 893.3333333333334, 966.6666666666667, 893.3333333333334, 766.6666666666667, 833.3333333333334, 973.3333333333334, 1006.6666666666667, 1193.3333333333335, 1006.6666666666667, 940.0, 1046.6666666666667, 966.6666666666667, 1173.3333333333335, 966.6666666666667, 1126.6666666666667, 1200.0, 1100.0, 1120.0, 1113.3333333333335, 1200.0, 1280.0, 1186.6666666666667, 1246.6666666666667, 1560.0, 1460.0, 1580.0, 1406.6666666666667, 1606.6666666666667, 1406.6666666666667, 1526.6666666666667, 1660.0, 1686.6666666666667, 1800.0, 1946.6666666666667, 1906.6666666666667, 1726.6666666666667, 1740.0, 1773.3333333333335, 1700.0, 1613.3333333333335, 1720.0, 1520.0, 1480.0, 1386.6666666666667, 1600.0, 1540.0, 1433.3333333333335, 1346.6666666666667, 1173.3333333333335, 1153.3333333333335, 1206.6666666666667, 1300.0, 1193.3333333333335, 1393.3333333333335, 1213.3333333333335, 960.0, 1066.6666666666667, 1146.6666666666667, 1200.0, 1086.6666666666667, 1046.6666666666667, 1020.0, 980.0, 913.3333333333334, 1033.3333333333335, 1020.0, 800.0, 1013.3333333333334, 966.6666666666667, 813.3333333333334, 873.3333333333334, 1033.3333333333335, 786.6666666666667, 900.0, 826.6666666666667, 793.3333333333334, 1046.6666666666667, 906.6666666666667, 986.6666666666667, 1100.0, 1033.3333333333335, 1126.6666666666667, 960.0, 933.3333333333334, 1006.6666666666667, 1013.3333333333334, 933.3333333333334, 826.6666666666667, 1066.6666666666667, 853.3333333333334, 793.3333333333334, 880.0, 880.0, 1053.3333333333335, 886.6666666666667, 960.0, 853.3333333333334, 960.0, 886.6666666666667, 993.3333333333334, 986.6666666666667, 926.6666666666667, 1013.3333333333334, 1160.0, 1006.6666666666667, 960.0], [0.0, 0.0, 0.0, 0.0, 0.0, 0.0, 0.0, 0.0, 0.0, 0.0, 0.0, 0.0, 0.0, 0.0, 0.0, 0.0, 0.0, 0.0, 0.0, 0.0, 0.0, 0.0, 0.0, 0.0, 0.0, 0.0, 0.0, 0.0, 0.0, 0.0, 0.0, 0.0, 0.0, 0.0, 0.0, 0.0, 0.0, 0.0, 0.0, 0.0, 0.0, 0.0, 0.0, 0.0, 0.0, 0.0, 0.0, 0.0, 0.0, 0.0, 0.0, 0.0, 0.0, 0.0, 0.0, 0.0, 0.0, 0.0, 0.0, 0.0, 0.0, 0.0, 0.0, 0.0, 0.0, 0.0, 0.0, 0.0, 0.0, 0.0, 0.0, 0.0, 0.0, 0.0, 0.0, 0.0, 0.0, 0.0, 0.0, 0.0, 0.0, 0.0, 0.0, 0.0, 0.0, 0.0, 0.0, 0.0, 0.0, 0.0, 0.0, 0.0, 0.0, 0.0, 0.0, 0.0, 0.0, 0.0, 0.0, 0.0, 0.0, 0.0, 0.0, 0.0, 0.0, 0.0, 0.0, 0.0, 0.0, 0.0, 0.0, 0.0, 0.0, 0.0, 0.0, 0.0, 0.0, 0.0, 0.0, 0.0, 0.0, 0.0, 0.0, 0.0, 0.0, 0.0, 0.0, 0.0, 0.0, 0.0, 0.0, 0.0, 0.0, 0.0, 0.0, 0.0, 0.0, 0.0, 0.0, 0.0, 0.0, 0.0, 0.0, 0.0, 0.0, 0.0, 0.0, 0.0, 0.0, 0.0, 0.0, 0.0, 0.0, 0.0, 0.0, 0.0, 0.0, 0.0, 0.0, 0.0, 0.0, 0.0, 0.0, 0.0, 0.0, 0.0, 0.0, 0.0, 0.0, 0.0, 0.0, 0.0, 0.0, 0.0, 0.0, 0.0, 0.0, 0.0, 0.0, 0.0, 0.0, 0.0, 0.0, 0.0, 0.0, 0.0, 0.0, 0.0, 0.0, 0.0, 0.0, 0.0, 0.0, 0.0, 0.0, 0.0, 0.0, 0.0, 0.0, 0.0, 0.0, 0.0, 0.0, 0.0, 0.0, 0.0, 0.0, 0.0, 0.0, 0.0, 0.0, 0.0, 0.0, 0.0, 0.0, 0.0, 0.0, 0.0, 0.0, 0.0, 0.0, 0.0, 0.0, 0.0, 0.0, 0.0, 0.0, 0.0, 0.0, 0.0, 0.0, 0.0, 0.0, 0.0, 0.0, 0.0, 0.0, 0.0, 0.0, 0.0, 0.0, 0.0, 0.0, 0.0, 0.0, 0.0, 0.0, 0.0, 0.0, 0.0, 0.0, 0.0, 0.0, 0.0, 0.0, 0.0, 0.0, 0.0, 0.0, 0.0, 0.0, 0.0, 0.0, 0.0, 0.0, 0.0, 0.0, 0.0, 0.0, 0.0, 0.0, 0.0, 0.0, 0.0, 0.0, 0.0, 0.0, 0.0, 0.0, 0.0, 0.0, 0.0, 0.0, 0.0, 0.0, 0.0, 0.0, 0.0, 0.0, 0.0, 0.0, 0.0, 0.0, 0.0, 0.0, 0.0, 0.0, 0.0, 0.0, 0.0, 0.0, 0.0, 0.0, 0.0, 0.0, 0.0, 0.0, 0.0, 0.0, 0.0, 0.0, 0.0, 0.0, 0.0, 0.0, 0.0, 0.0, 0.0, 0.0, 0.0, 0.0, 0.0, 0.0, 0.0, 0.0, 0.0, 0.0, 0.0, 0.0, 0.0, 0.0, 0.0, 0.0, 0.0, 0.0, 0.0, 0.0, 0.0, 0.0, 0.0, 0.0, 0.0, 0.0, 0.0, 0.0, 0.0, 0.0, 0.0, 0.0, 0.0, 0.0, 0.0, 0.0, 0.0, 0.0, 0.0, 0.0, 0.0, 0.0, 0.0, 0.0, 0.0, 0.0, 0.0, 0.0, 0.0, 0.0, 0.0, 0.0, 0.0, 0.0, 0.0, 0.0, 0.0, 0.0, 0.0, 0.0, 0.0, 0.0, 0.0, 0.0, 0.0, 0.0, 0.0, 0.0, 0.0, 0.0, 0.0, 0.0, 0.0, 0.0, 0.0, 0.0, 0.0, 0.0, 0.0, 0.0, 0.0, 0.0, 0.0, 0.0, 0.0, 0.0, 0.0, 0.0, 0.0, 0.0, 0.0, 0.0, 0.0, 0.0, 0.0, 0.0, 0.0, 0.0, 0.0, 0.0, 0.0, 0.0, 0.0, 0.0, 0.0, 0.0, 0.0, 0.0, 0.0, 0.0, 0.0, 0.0, 0.0, 0.0, 0.0, 0.0, 0.0, 0.0, 0.0, 0.0, 0.0, 0.0, 0.0, 0.0, 0.0, 0.0, 0.0, 0.0, 0.0, 0.0, 0.0, 0.0, 0.0, 0.0, 0.0, 0.0, 0.0, 0.0, 0.0, 0.0, 0.0, 0.0, 0.0, 0.0, 0.0, 0.0, 0.0, 0.0, 0.0, 0.0, 0.0, 0.0, 0.0, 0.0, 0.0, 0.0, 0.0, 0.0, 0.0, 0.0, 0.0, 0.0, 0.0, 0.0, 0.0, 0.0, 0.0, 0.0, 0.0, 0.0, 0.0, 0.0, 0.0, 0.0, 0.0, 0.0, 0.0, 0.0, 0.0, 0.0, 0.0, 0.0, 0.0, 0.0, 0.0, 0.0, 0.0, 0.0, 0.0, 0.0, 0.0, 0.0, 0.0, 0.0, 0.0, 0.0, 0.0, 0.0, 0.0, 0.0, 0.0, 0.0, 0.0, 0.0, 0.0, 0.0, 0.0, 0.0, 0.0, 0.0, 0.0, 0.0, 0.0, 0.0, 0.0, 0.0, 0.0, 0.0, 0.0, 0.0, 0.0, 0.0, 0.0, 0.0, 0.0, 0.0, 0.0, 0.0, 0.0, 0.0, 0.0, 0.0, 0.0, 0.0, 0.0, 0.0, 0.0, 0.0, 0.0, 0.0, 0.0, 0.0, 0.0, 0.0, 0.0, 0.0, 0.0, 0.0, 0.0, 0.0, 0.0, 0.0, 0.0, 0.0, 0.0, 0.0, 0.0, 0.0, 0.0, 0.0, 0.0, 0.0, 0.0, 0.0, 0.0, 0.0, 0.0, 0.0, 0.0, 0.0, 0.0, 0.0, 0.0, 0.0, 0.0, 0.0, 0.0, 0.0, 0.0, 0.0, 0.0, 0.0, 0.0, 0.0, 0.0, 0.0, 0.0, 0.0, 0.0, 0.0, 0.0, 0.0, 0.0, 0.0, 0.0, 0.0, 0.0, 0.0, 0.0, 0.0, 0.0, 0.0, 0.0, 0.0, 0.0, 0.0, 0.0, 0.0, 0.0, 0.0, 0.0, 0.0, 0.0, 0.0, 0.0, 0.0, 0.0, 0.0, 0.0, 0.0, 0.0, 0.0, 0.0, 0.0, 0.0, 0.0, 0.0, 0.0, 0.0, 0.0, 0.0, 0.0, 0.0, 0.0, 0.0, 0.0, 0.0, 0.0, 0.0, 0.0, 0.0, 0.0, 0.0, 0.0, 0.0, 0.0, 0.0, 0.0, 0.0, 0.0, 0.0, 0.0, 0.0, 0.0, 0.0, 0.0, 0.0, 0.0, 0.0, 0.0, 0.0, 0.0, 0.0, 0.0, 0.0, 0.0, 0.0, 0.0, 0.0, 0.0, 0.0, 0.0, 0.0, 0.0, 0.0, 0.0, 0.0, 0.0, 0.0, 0.0, 0.0, 0.0, 0.0, 0.0, 0.0, 0.0, 0.0, 0.0, 0.0, 0.0, 0.0, 0.0, 0.0, 0.0, 0.0, 0.0, 0.0, 0.0, 0.0, 0.0, 0.0, 0.0, 0.0, 0.0, 0.0, 0.0, 0.0, 0.0, 0.0, 0.0, 0.0, 0.0, 0.0, 0.0, 0.0, 0.0, 0.0, 0.0, 0.0, 0.0, 0.0, 0.0, 0.0, 0.0, 0.0, 0.0, 0.0, 0.0, 0.0, 0.0, 0.0, 0.0, 0.0, 0.0, 0.0, 0.0, 0.0, 0.0, 0.0, 0.0, 0.0, 0.0, 0.0, 0.0, 0.0, 0.0, 0.0, 0.0, 0.0, 0.0, 0.0, 0.0, 0.0, 0.0, 0.0, 0.0, 0.0, 0.0, 0.0, 0.0, 0.0, 0.0, 0.0, 0.0, 0.0, 0.0, 0.0, 0.0, 0.0, 0.0, 0.0, 0.0, 0.0, 0.0, 0.0, 0.0, 0.0, 0.0, 0.0, 0.0, 0.0, 0.0, 0.0, 0.0, 0.0, 0.0, 0.0, 0.0, 0.0, 0.0, 0.0, 0.0, 0.0, 0.0, 0.0, 0.0, 0.0, 0.0, 0.0, 0.0, 0.0, 0.0, 0.0, 0.0, 0.0, 0.0, 0.0, 0.0, 0.0, 0.0, 0.0, 0.0, 0.0, 0.0, 0.0, 0.0, 0.0, 0.0, 0.0, 0.0, 0.0, 0.0, 0.0, 0.0, 0.0, 0.0, 0.0, 0.0, 0.0, 0.0, 0.0, 0.0, 0.0, 0.0, 0.0, 0.0, 0.0, 0.0, 0.0, 0.0, 0.0, 0.0, 0.0, 0.0, 0.0, 0.0, 0.0, 0.0, 0.0, 0.0, 0.0, 0.0, 0.0, 0.0, 0.0, 0.0, 0.0, 0.0, 0.0, 0.0, 0.0, 0.0, 0.0, 0.0, 0.0, 0.0, 0.0, 0.0, 0.0, 0.0, 0.0, 0.0, 0.0, 0.0, 0.0, 0.0, 0.0, 0.0, 0.0, 0.0, 0.0, 0.0, 0.0, 0.0, 0.0, 0.0, 0.0, 0.0, 0.0, 0.0, 0.0, 0.0, 0.0, 0.0, 0.0, 0.0, 0.0, 0.0, 0.0, 0.0, 0.0, 0.0, 0.0, 0.0, 0.0, 0.0, 0.0, 0.0, 0.0, 0.0, 0.0, 0.0, 0.0, 0.0, 0.0, 0.0, 0.0, 0.0, 0.0, 0.0, 0.0, 0.0, 0.0, 0.0, 0.0, 0.0, 0.0, 0.0, 0.0, 0.0, 0.0, 0.0, 0.0, 0.0, 0.0, 0.0, 0.0, 0.0, 0.0, 0.0, 0.0, 0.0, 0.0, 0.0, 0.0, 0.0, 0.0, 0.0, 0.0, 0.0, 0.0, 0.0, 0.0, 0.0, 0.0, 0.0, 0.0, 0.0, 0.0, 0.0, 0.0, 0.0, 0.0, 0.0, 0.0]] caption="Most Recent Time Trace"
